vi "Robot Global Data.vi"() -> ()   [LabVIEW 2016]
doc: "This global VI can contain as many global variables as you need. Place a control on the panel, give it a good name. To read or write to it from a VI, drag the icon to the diagram of that VI. You can also drag from the project. Click on the node to change which global you access. You shouldn't have multiple locations writing to a global or it will cause a race-condition."
uses:
  <vilib>/Rock Robotics/WPI/Camera/WPI_CameraImageSize.ctl
  <vilib>/Rock Robotics/WPI/DriverStation/WPI_DriverStationRobotMode2.ctl
panel:
  out "LED: Turbo":bool
  out "LED: Gear":bool
  out "LED: Shoot":bool
  out "LED: Hang":bool
  out "LED: Low Gear":bool
  out "Gear Deployed":bool
  out "Manipulator On":bool
  out "Shooter P":dbl
  out "Disabled":bool
  in  "Shooter Speed Setpoint":dbl
  in  "Shooter Speed":dbl(slide) scale=0.0..1.0
  in  "LED State":i8
  out "Eject Gear":bool
  out "Drive Encoder Distance":dbl
  out "Selected Auto Path":path
  in  "Zero Yaw?":bool
  out "Robot Yaw Offset":dbl
  out "Robot Yaw":dbl
  out "Right Drive Speed":dbl
  out "Left Drive Speed":dbl
  in  "Robot Mode":T1
  in  "image size":T2=enum."320x240"
  in  "Enable Vision":bool
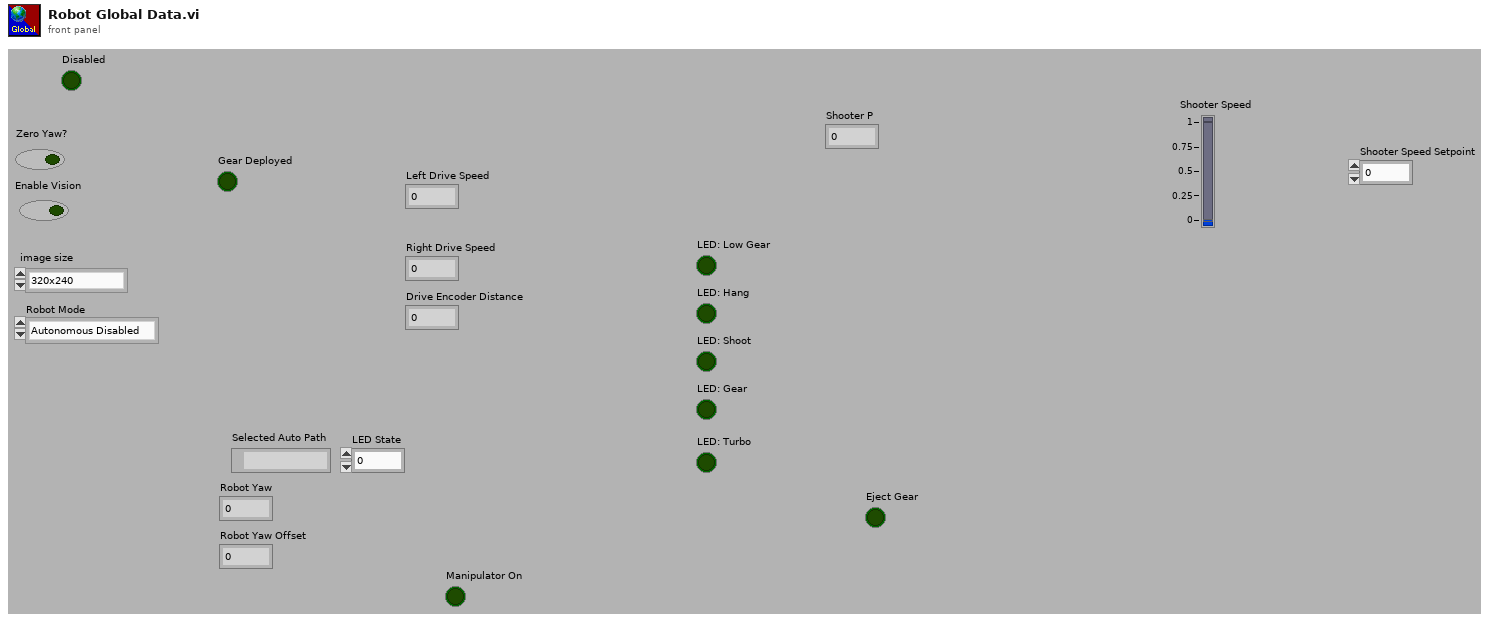
[diagram p1: front panel]
types:
  T1 = typedef "WPI_DriverStationRobotMode2.ctl" = enum16{"Autonomous Disabled", "Autonomous Enabled", "Teleop Disabled", "Teleop Enabled", "Disconnected", "Finish", "Test Disabled", "Test Enabled", "Emergency Stopped"}
  T2 = typedef "WPI_CameraImageSize.ctl" = enum16{"640x480", "320x240", "160x120", "Custom"}
diagram:
